vi "control.vi"() -> ()   [LabVIEW 2010]
uses:
  <vilib>/sound2/lvsound2.llb/Sound Data Format.ctl
  <vilib>/addons/PixeLINK/Low Level Functions/CAMERA_FEATURES.llb/TDPU-CameraFeatures-PixelFormat.ctl
  <vilib>/sound2/lvsound2.llb/Sound Output Task ID.ctl
  <vilib>/vision/Image Controls.llb/IMAQ Image.ctl
panel:
  out "time (ms)":u32
  out "Contraste":dbl(graph)
  out "Todo Funciona?":bool
  out "Waveform DAQ":waveform(dbl)(graph)
  out "Image":T1(plugin-control)
  in  "Tab Control":enum32{"DAQ", "Sound", "Camara", "Control"}(tab)
  in  "Calibracion DAQ":T2
  in  "DAQ Controls":T3={"Minimum Value"=-10.0, "Maximum Value"=10.0, "Physical Channel"="Dev1/ao0", "DAQ Fs (S/s)"=10000.0} {"Minimum Value" min=-10.0 max=0.0; "Maximum Value" min=0.0 max=10.0}
  in  "DAQ?":bool
  in  "Sound Controls":T5={"device ID"=0, "sound format"={"sample rate (S/s)"=44000.0, "number of channels"=2, "bits per sample"=16}, "time (ms)"=200.0}
  in  "Sound?":bool
  in  "Frecuencia":dbl
  in  "Selector":u16(ring) items=["776002034"]
  in  "Streeam?":bool
  in  "Camera Parameters":T7 {"Pixel Format" items=["PIXEL_FORMAT_MONO8", "PIXEL_FORMAT_MONO16", "PIXEL_FORMAT_YUV422", "PIXEL_FORMAT_BAYER8_GRBG", "PIXEL_FORMAT_BAYER16_GRBG", "PIXEL_FORMAT_RGB24", "PIXEL_FORMAT_RGB48", "PIXEL_FORMAT_BAYER8_RGGB", "PIXEL_FORMAT_BAYER8_GBRG ", "PIXEL_FORMAT_BAYER8_BGGR ", "PIXEL_FORMAT_BAYER16_RGGB ", "PIXEL_FORMAT_BAYER16_GBRG", "PIXEL_FORMAT_BAYER16_BGGR", "PIXEL_FORMAT_RGB32"]}
  out "Camara Funciona?":bool
  out "Contraste":dbl
  in  "Control Parameters":T8={"N Init Avg"=6, "N Avg Best"=3, "% Best to test"=0.95, "% Best to beat"=1.0}
  in  "lamda (nm)":dbl=546.1
  in  "Reset Control":bool
  in  "Control ON?":bool
  in  "Ajuste ON?":bool
  in  "stop":bool
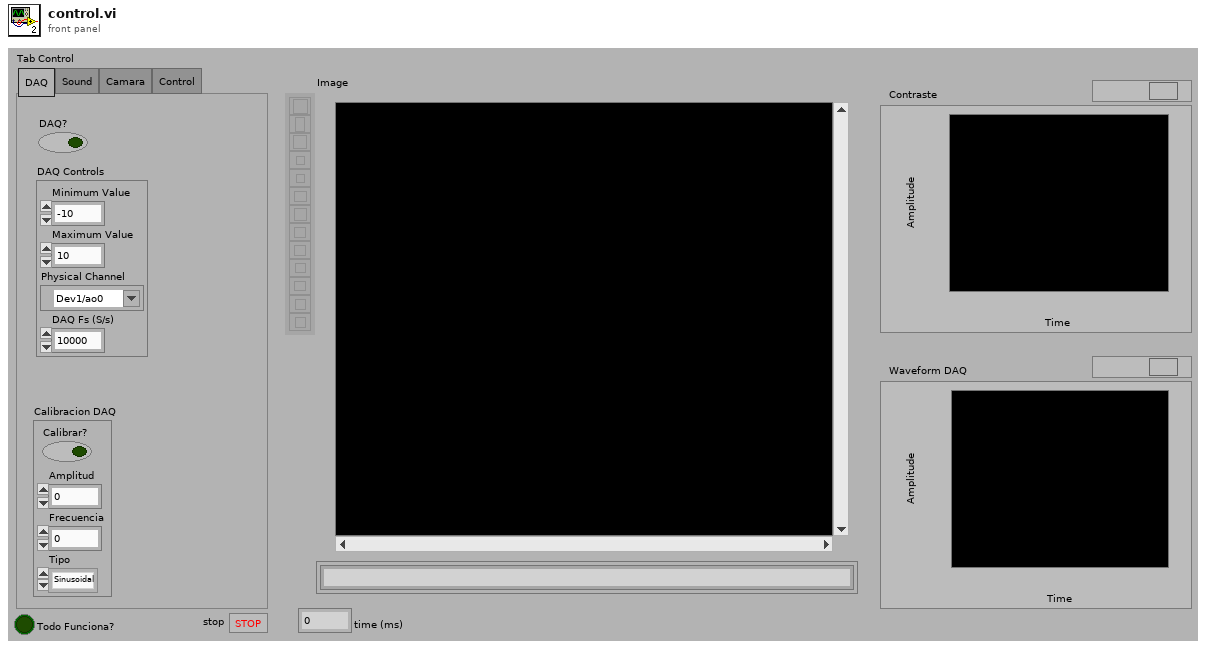
[diagram p1: front panel]
types:
  T1 = typedef "IMAQ Image.ctl" = refnum<image>
  T2 = cluster{"Calibrar?":bool, "Amplitud":dbl, "Frecuencia":dbl, "Tipo":enum16{"Sinusoidal", "Triangular", "Cuadrada"}}
  T3 = cluster{"Minimum Value":dbl, "Maximum Value":dbl, "Physical Channel":tag, "DAQ Fs (S/s)":dbl}
  T4 = typedef "Sound Data Format.ctl" = cluster{"sample rate (S/s)":dbl, "number of channels":i32, "bits per sample":i32}
  T5 = cluster{"device ID":u32, "sound format":T4, "time (ms)":dbl}
  T6 = typedef "TDPU-CameraFeatures-PixelFormat.ctl" = u16
  T7 = cluster{"Exposure Time (ms)":u32, "Gain (dB)":dbl, "Saturation (%)":dbl, "Brightness (%)":dbl, "Color Temperature":dbl, "ROI":cluster{"Top":i32, "Left":i32, "Width":i32, "Height":i32}, "White Balance Gain (dB)":cluster{"Red":dbl, "Green":dbl, "Blue":dbl}, "Gamma":dbl, "Pixel Format":T6}
  T8 = cluster{"N Init Avg":u32, "N Avg Best":u32, "% Best to test":dbl, "% Best to beat":dbl}
  T9 = cluster{"DAQ Fs (S/s)":dbl, "task":refnum<k21>, "error":errorcluster, "Min Value":dbl, "Max Value":dbl}
  T10 = cluster{"hCamera":u32, "Error":errorcluster, "uSerialNumber OUT":u32}
  T11 = typedef "Sound Output Task ID.ctl" = u32
  T12 = cluster{"task ID":T11, "error":errorcluster, "sound format":T4}
  T13 = cluster{"Amplitud":dbl, "Media":dbl, "Sigma":dbl}
  T14 = cluster{"hCamera":u32, "Error":errorcluster, "uSerialNumber":u32}
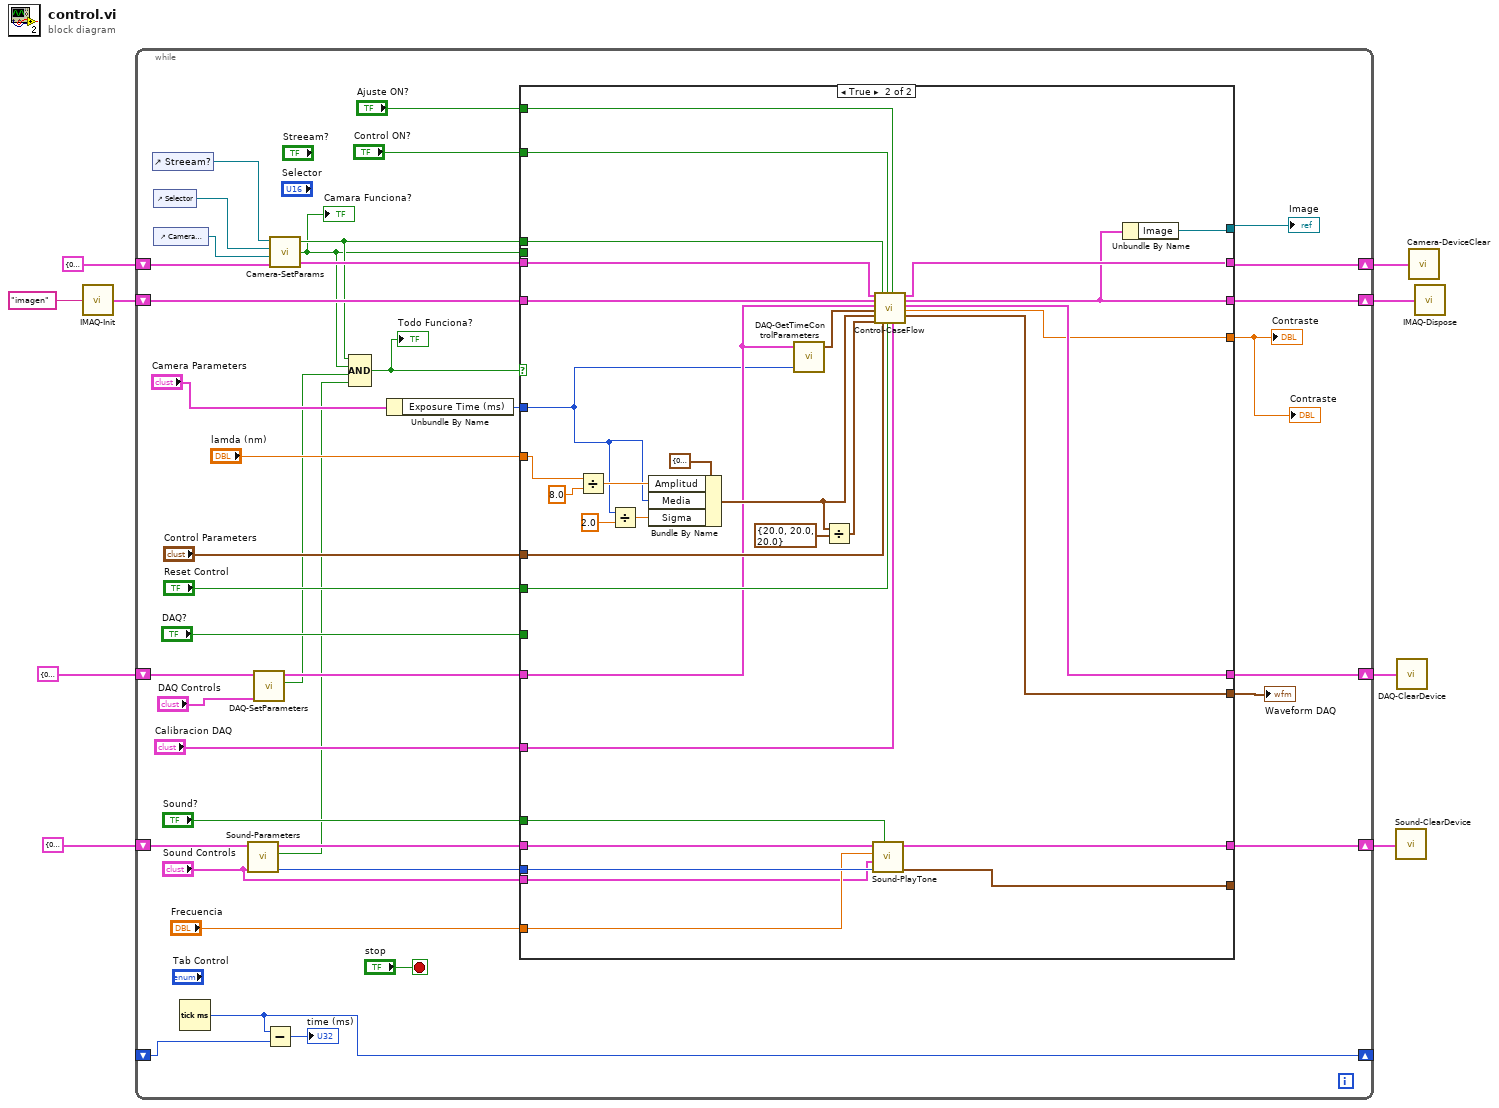
[diagram p0: block diagram]
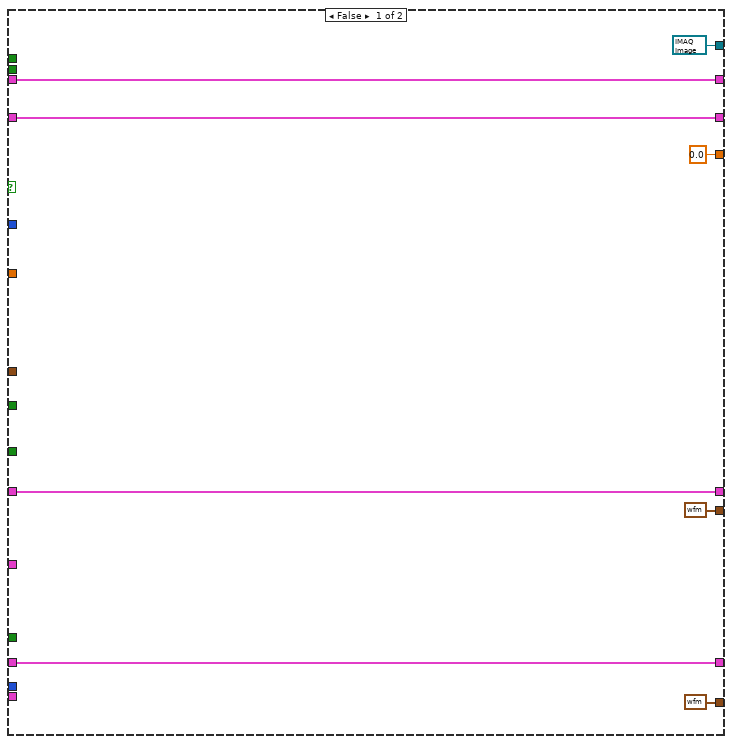
[diagram p2: hidden frame]
diagram:
  n1 = call "IMAQ-Init.vi"("Image Name"="imagen") -> ("Image Device IN"=w5:cluster{"Image":T1, "errorImage":errorcluster})
  n2 = while {
    shift-right: [w42] -> w7
    shift-left: T9 {"DAQ Fs (S/s)"=0.0, "task"="", "error"={"status"=FALSE, "code"=0, "source"=""}, "Min Value"=0.0, "Max Value"=0.0} ("DAQ Device OUT") -> [w43]
    shift-right: [w39] -> w8
    shift-left: T12 {"task ID"=0, "error"={"status"=TRUE, "code"=0, "source"=""}, "sound format"={"sample rate (S/s)"=0.0, "number of channels"=0, "bits per sample"=0}} ("Sound Device OUT") -> [w38]
    shift-right: [w26] -> w2
    shift-left: w5 -> [w30]
    shift-right: [w29] -> w3
    shift-left: T10 {"hCamera"=0, "Error"={"status"=FALSE, "code"=0, "source"=""}, "uSerialNumber OUT"=0} ("Camera Device  IN") -> [w28]
    shift-right: [w12] -> _
    shift-left: _ -> [w11]
    stop <- "stop" stop-if-true
    n3 = control-ref of="Streeam?"() -> (w32:refnum<vi>)
    n4 = control-ref of="Selector"() -> (w34:refnum<vi>)
    n5 = control-ref of="Camera Parameters"() -> (w33:refnum<vi>)
    n6 = Tick Count (ms)() -> (millisecond timer value=w12:u32)
    n7 = call "Sound-Parameters.vi"("Sound Controls"="Sound Controls", "Sound Device IN"=w38) -> ("#samples"=w40:u32, "En funcionamiento?"=w14:bool, "Sound Device OUT"=w41:T12)  [unwired: 3 in]
    n8 = call "DAQ-SetParameters.vi"("DAQ Controls"="DAQ Controls", "DAQ Device IN"=w43) -> ("En Funcionamiento?"=w15:bool, "DAQ Device OUT"=w47:T9)  [unwired: 4 in]
    n9 = Subtract(x=w12, y=w11) -> (x-y=→"time (ms)":u32)
    n10 = call "Camera-SetParams.vi"("Camera Device  IN"=w28, "Camera Parameters"=w33, "Selector"=w34, "Stream?"=w32) -> ("Camera Device OUT"=w31:T14, "Funciona?"=w16:bool, "Stream? OUT"=w17:bool)
    "Camara Funciona?" <- w16
    n11 = Compound Arithmetic op=AND(w17, w16, w15, w14) -> (w18:bool)
    "Todo Funciona?" <- w18
    n12 = Unbundle By Name("Camera Parameters") -> ("Exposure Time (ms)"=w21:u32)
    n13 = case shown="True" w18 {
      tunnel: "DAQ?" -> [_ _]
      tunnel: w47 -> [w54 w66]
      tunnel: [waveform(dbl) {"t0"=timestamp(0 s since 1904-01-01), "dt"=1.0, "Y"=[]} ("Waveform") w59] -> w46
      tunnel: "Calibracion DAQ" -> [_ w67]
      tunnel: [w54 w80] -> w42
      tunnel: [waveform(dbl) {"t0"=timestamp(0 s since 1904-01-01), "dt"=1.0, "Y"=[]} ("Waveform") w90] -> _
      tunnel: w41 -> [w51 w89]
      tunnel: w40 -> [_ w88]
      tunnel: [w51 w87] -> w39
      tunnel: "Sound?" -> [_ w86]
      tunnel: "Frecuencia" -> [_ w85]
      tunnel: "Sound Controls" -> [_ w84]
      tunnel: w31 -> [w56 w83]
      tunnel: w30 -> [w55 w81]
      tunnel: [w56 w82] -> w29
      tunnel: [T1 refnum ("Image") w61] -> w27
      tunnel: [w55 w60] -> w26
      tunnel: [0.0 ("Contraste") w79] -> w13
      tunnel: w16 -> [_ _]
      tunnel: w17 -> [_ w64]
      tunnel: "lamda (nm)" -> [_ w72]
      tunnel: w21 -> [_ w58]
      tunnel: "Control Parameters" -> [_ w69]
      tunnel: "Reset Control" -> [_ w68]
      tunnel: "Ajuste ON?" -> [_ w63]
      tunnel: "Control ON?" -> [_ w62]
      frame False {
      }
      frame True {
        n14 = Divide(x=w72, y=8.0) -> (x/y=w74:dbl)
        n15 = Divide(x=w58, y=2.0) -> (x/y=w77:dbl)
        n16 = Bundle By Name(cluster=T13 {"Amplitud"=0.0, "Media"=0.0, "Sigma"=0.0} ("Parametros Maximos"), "Amplitud"=w74, "Media"=w58, "Sigma"=w77) -> (w71:T13)
        n17 = call "DAQ-GetTimeControlParameters.vi"("tiempo (ms)"=w58, "DAQ Device IN"=w66) -> ("Time Control Parameters"=w78:cluster{"# samples":u32, "tiempos (ms)":dbl})  [unwired: 2 in, 1 out]
        n18 = Divide(x=w71, y=T13 {"Amplitud"=20.0, "Media"=20.0, "Sigma"=20.0}) -> (x/y=w70:T13)
        n19 = call "Sound-PlayTone.vi"("sound?"=w86, "# samples"=w88, "Sound Controls"=w84, "Frecuencia"=w85, "Sound Device IN"=w89) -> ("Waveform"=w90:waveform(dbl), "Sound Device OUT"=w87:T12)  [unwired: 3 in]
        n20 = call "Control-CaseFlow.vi"("Camera Device  IN"=w83, "Image Device IN"=w81, "DAQ Device IN"=w66, "Time Control Parameters"=w78, "Parametros Maximos"=w71, "detla Parametros"=w70, "Camara ON?"=w64, "Control Parameters"=w69, "Control?"=w62, "Reset Control"=w68, "Ajuste?"=w63, "Calibracion DAQ"=w67) -> ("Camera Device OUT"=w82:T10, "Image Device OUT"=w60:cluster{"Image":T1, "errorImage":errorcluster}, "DAQ Device OUT"=w80:T9, "Contraste"=w79:dbl, "Waveform"=w59:waveform(dbl))  [unwired: 2 in, 1 out]
        n21 = Unbundle By Name(w60) -> ("Image"=w61:T1)
      }
    }
    "Waveform DAQ" <- w46
    "Image" <- w27
    "Contraste" <- w13
    "Contraste" <- w13
  }
  n22 = call "Sound-ClearDevice.vi"("Sound Device OUT"=w8) -> ()
  n23 = call "DAQ-ClearDevice.vi"("DAQ Device IN"=w7) -> ()
  n24 = call "Camera-DeviceClear.vi"("Camera Device OUT"=w3) -> ()
  n25 = call "IMAQ-Dispose.vi"("Image Device IN"=w2) -> ()
